vi "XYZ Ultrasonic Scanning Software v1.3 (Movement).vi"() -> ()   [LabVIEW 2020]
uses:
  <instrlib>/Arcus Ethernet Driver 1.0.0/ArcusEthernetComm/classes/Controller/_Controller.lvclass
panel:
  in  "Tab Control":T1(tab)
  in  "Check Rig Connection":bool
  out "Succesful Rig Connection":bool=TRUE
  in  "Error In":errorcluster
  in  "Move Y Distance":dbl
  in  "Set Starting Position":bool
  in  "Z Direction":bool=TRUE
  in  "Y Direction":bool=TRUE
  in  "Move X Distance":dbl
  in  "Move Z Distance":dbl
  in  "X Direction":bool=TRUE
  in  "Return To Home":bool
  in  "Move":bool
  in  "Start A-Scan":bool
  in  "Start B-Scan":bool
  in  "Initial X Direction":bool=TRUE
  in  "Initial Y Direction":bool=TRUE
  in  "Initial Z Direction":bool=TRUE
  in  "Confirm Scanning Parameters B-Scan":bool
  in  "Height (mm)":dbl
  in  "Width (mm)":dbl
  in  "Length (mm)":dbl
  in  "Select Axis To Scan":enum32{"No Selection", "X", "Y", "Z"}(radio)
  in  "Scan C-Scan":bool
  in  "Length (mm)":dbl
  in  "Width (mm)":dbl
  in  "Height (mm)":dbl
  in  "Confirm Dimensions":bool
  in  "Initial X Direction":bool=TRUE
  in  "Initial Y Direction":bool=TRUE
  in  "Initial Z Direction":bool=TRUE
  in  "Select Plane To Scan":enum32{"No Selection", "XY", "XZ", "YZ"}(radio)
  # "Moving To Starting Point (mm)"
  # "Scanning Parameters"
  # "Tank Dimensions"
  # "Y - Width"
  # "X - Length"
  # "Z - Height"
  # "Scanning Parameters"
  # "Tank Dimensions"
  # "Y - Width"
  # "X - Length"
  # "Z - Height"
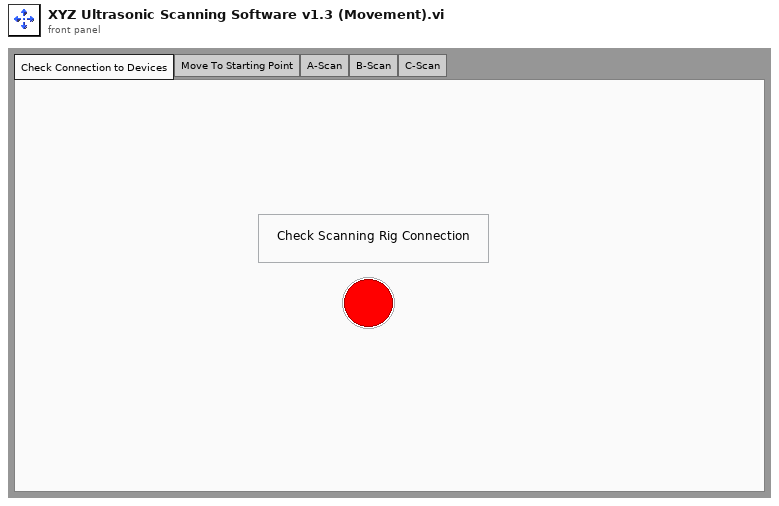
[diagram p1: front panel]
types:
  T1 = enum32{"Check Connection to Devices", "Move To Starting Point", "A-Scan", "B-Scan", "C-Scan"}
  T2 = enum8{"Enabled", "Disabled", "Disabled and Grayed Out"}
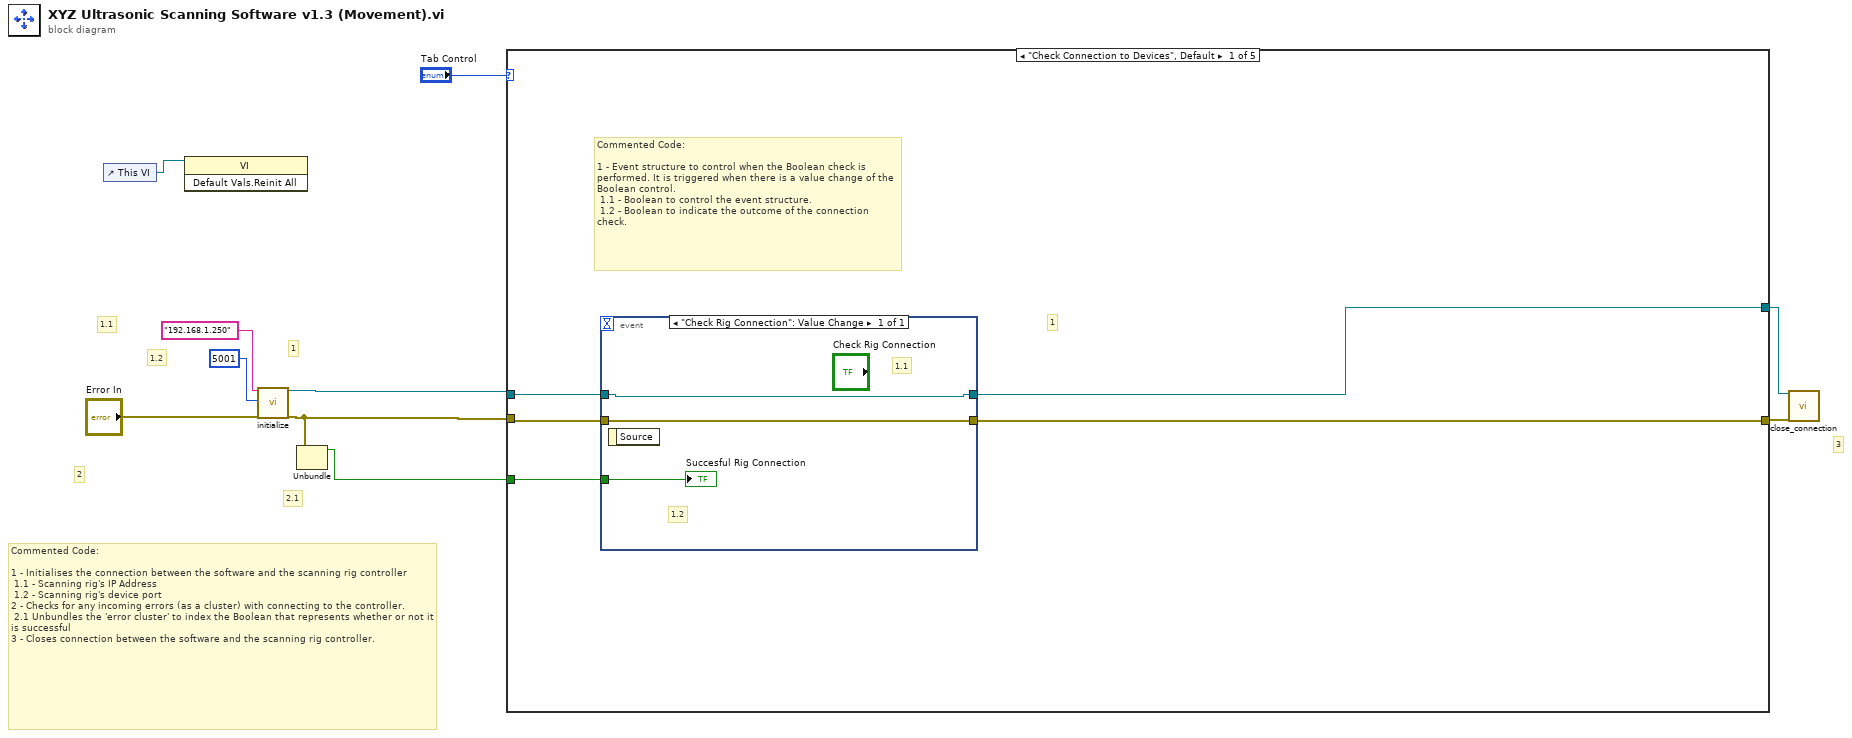
[diagram p0: block diagram]
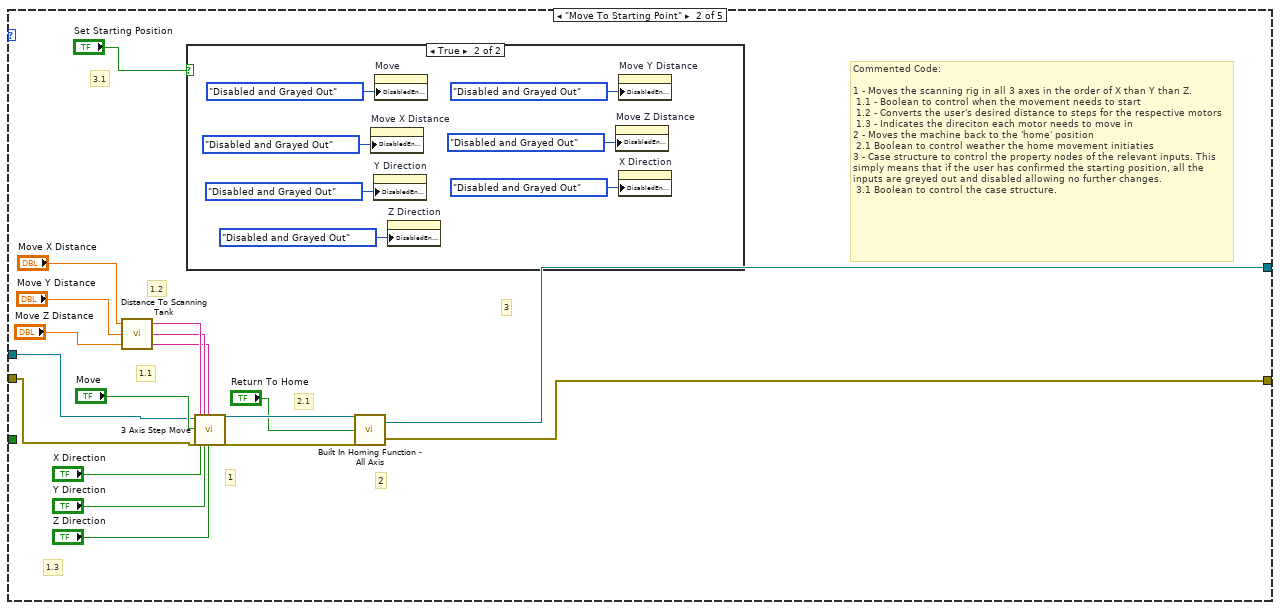
[diagram p2: hidden frame]
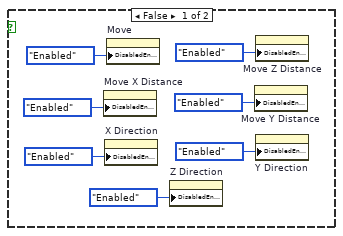
[diagram p3: hidden frame]
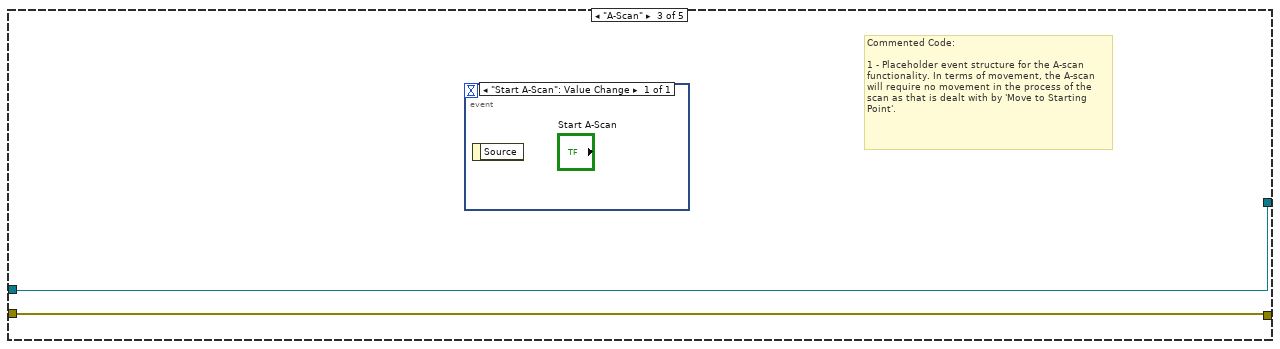
[diagram p4: hidden frame]
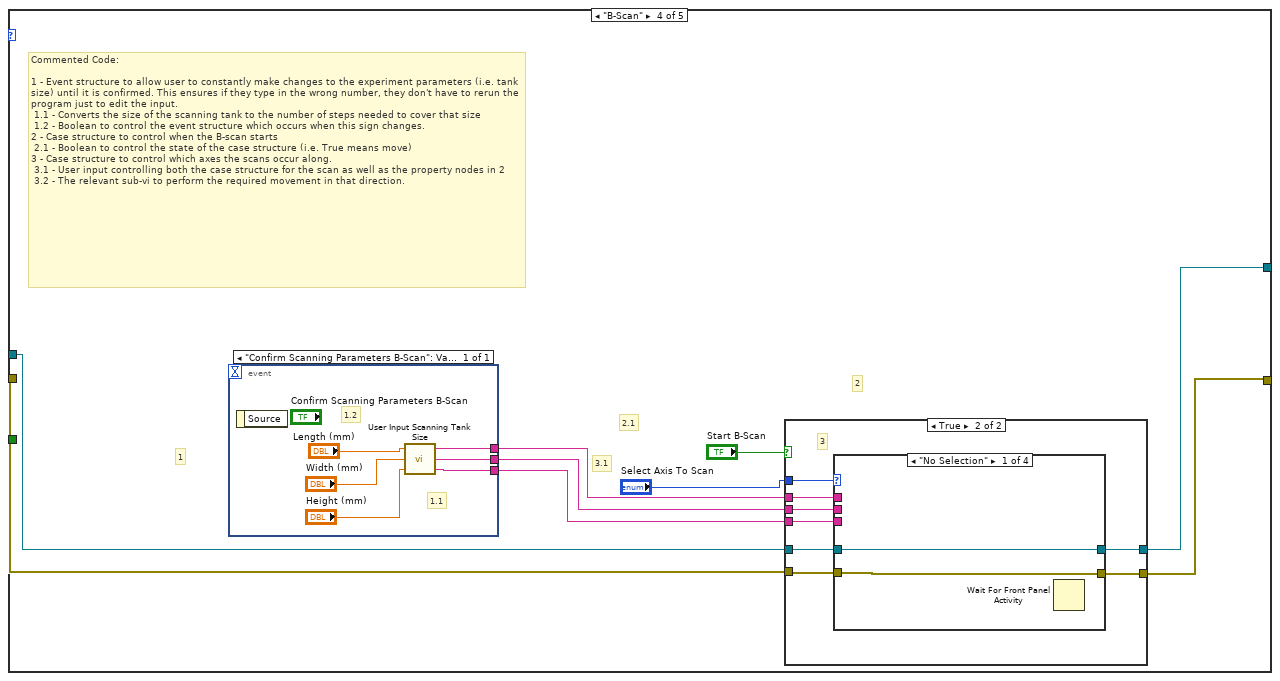
[diagram p5: hidden frame]
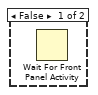
[diagram p6: hidden frame]
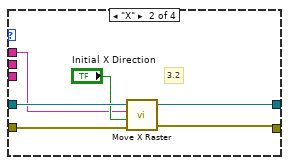
[diagram p7: hidden frame]
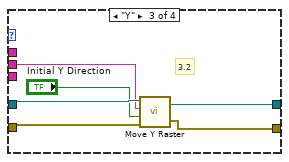
[diagram p8: hidden frame]
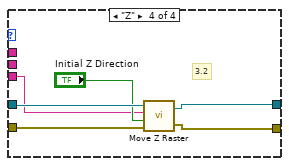
[diagram p9: hidden frame]
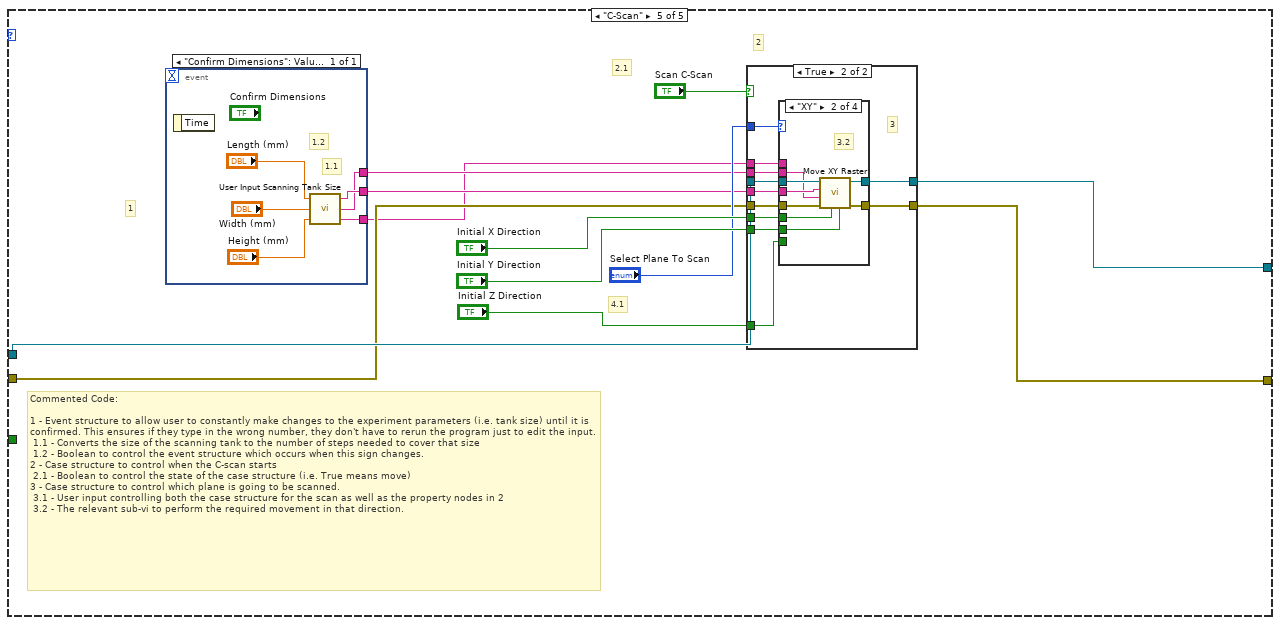
[diagram p10: hidden frame]
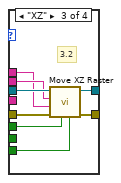
[diagram p13: hidden frame]
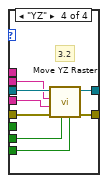
[diagram p14: hidden frame]
diagram:
  # "3"
  # "2"
  # "2.1"
  # "1.2"
  # "1.1"
  # "1"
  # "Commented Code:\n\n1 - Initialises the connection between the software and the scanning rig controller\n 1.1 - Scanning rig's IP Address\n 1.2 - Scanning rig's device port\n2 - Checks for any incoming errors (as a cluster) with connecting to the controller.  \n 2.1 Unbundles the 'error cluster' to index the Boolean that represents whether or not it is successful\n3 - Closes connection between the software and the scanning rig controller."
  n1 = control-ref of="This VI"() -> (w3:refnum<vi>)
  n2 = invoke class="VI" method="Default Vals.Reinit All"(reference=w3) -> ()  [unwired: 2 in, 3 out]
  n3 = call <instrlib>:"initialize.vi"("ip_address (in)"="192.168.1.250", "dev_port(def=5001)"=u16 5001, "error in (no error)"="Error In") -> ("reference (out)"=w9:refnum<class "_Controller.lvclass">, "error out"=w10:errorcluster)  [unwired: 15 in]
  n4 = Unbundle(w10) -> ("status"=w1:bool)  [unwired: 2 out]
  n5 = case shown="\"Check Connection to Devices\", Default" "Tab Control" {
    tunnel: w9 -> [w15 w26 w52 w60 w104]
    tunnel: [w13 w21 w52 w55 w103] -> w5
    tunnel: [w12 w22 w51 w53 w102] -> w4
    tunnel: w10 -> [w14 w25 w51 w59 w99]
    tunnel: w1 -> [w11 _ _ _ _]
    frame "Check Connection to Devices", Default {
      # "1"
      # "Commented Code:\n\n1 - Event structure to control when the Boolean check is performed. It is triggered when there is a value change of the Boolean control. \n 1.1 - Boolean to control the event structure. \n 1.2 - Boolean to indicate the outcome of the connection check."
      n6 = event shown="[0] \"Check Rig Connection\": Value Change" {
        selector: _ -> [_]
        dyn-events: _ -> [_]
        timeout: _ -> [_]
        tunnel: w15 -> [w18]
        tunnel: w14 -> [w17]
        tunnel: [w18] -> w13
        tunnel: [w17] -> w12
        tunnel: w11 -> [w16]
        event "Check Rig Connection": Value Change {
          # "1.1"
          # "1.2"
          n7 = event-data() -> ()  [unwired: 1 in, 1 out]
          "Succesful Rig Connection" <- w16
        }
      }
    }
    frame "Move To Starting Point" {
      # "3.1"
      # "3"
      # "2.1"
      # "2"
      # "1.3"
      # "1.1"
      # "1"
      # "1.2"
      # "Commented Code:\n\n1 - Moves the scanning rig in all 3 axes in the order of X than Y than Z.\n 1.1 - Boolean to control when the movement needs to start\n 1.2 - Converts the user's desired distance to steps for the respective motors\n 1.3 - Indicates the direciton each motor needs to move in\n2 - Moves the machine back to the 'home' position\n 2.1 Boolean to control weather the home movement initiaties \n3 - Case structure to control the property nodes of the relevant inputs. This simply means that if the user has confirmed the starting position, all the inputs are greyed out and disabled allowing no further changes.\n 3.1 Boolean to control the case structure."
      n8 = call "Distance To Scanning Tank.vi"("Move Z Distance (mm)"="Move Z Distance", "Move Y Distance (mm)"="Move Y Distance", "Move X Distance (mm)"="Move X Distance") -> ("Z Steps"=w34:string, "Y Steps"=w35:string, "X Steps"=w36:string)
      n9 = case shown="True" "Set Starting Position" {
        frame False {
          n10 = property on="Move X Distance" class="DigNum (strict)"("DisabledEnum"=T2."Enabled" ("Disabled")) -> ()  [unwired: 2 in, 2 out]
          n11 = property on="X Direction" class="Bool (strict)"("DisabledEnum"=T2."Enabled" ("Disabled")) -> ()  [unwired: 2 in, 2 out]
          n12 = property on="Move" class="Bool"("DisabledEnum"=T2."Enabled" ("Disabled")) -> ()  [unwired: 2 in, 2 out]
          n13 = property on="Z Direction" class="Bool (strict)"("DisabledEnum"=T2."Enabled" ("Disabled")) -> ()  [unwired: 2 in, 2 out]
          n14 = property on="Move Y Distance" class="DigNum (strict)"("DisabledEnum"=T2."Enabled" ("Disabled")) -> ()  [unwired: 2 in, 2 out]
          n15 = property on="Move Z Distance" class="DigNum (strict)"("DisabledEnum"=T2."Enabled" ("Disabled")) -> ()  [unwired: 2 in, 2 out]
          n16 = property on="Y Direction" class="Bool (strict)"("DisabledEnum"=T2."Enabled" ("Disabled")) -> ()  [unwired: 2 in, 2 out]
        }
        frame True {
          n17 = property on="Move X Distance" class="DigNum (strict)"("DisabledEnum"=T2."Disabled and Grayed Out" ("Disabled")) -> ()  [unwired: 2 in, 2 out]
          n18 = property on="Y Direction" class="Bool (strict)"("DisabledEnum"=T2."Disabled and Grayed Out" ("Disabled")) -> ()  [unwired: 2 in, 2 out]
          n19 = property on="Move" class="Bool"("DisabledEnum"=T2."Disabled and Grayed Out" ("Disabled")) -> ()  [unwired: 2 in, 2 out]
          n20 = property on="Z Direction" class="Bool (strict)"("DisabledEnum"=T2."Disabled and Grayed Out" ("Disabled")) -> ()  [unwired: 2 in, 2 out]
          n21 = property on="Move Z Distance" class="DigNum (strict)"("DisabledEnum"=T2."Disabled and Grayed Out" ("Disabled")) -> ()  [unwired: 2 in, 2 out]
          n22 = property on="Move Y Distance" class="DigNum (strict)"("DisabledEnum"=T2."Disabled and Grayed Out" ("Disabled")) -> ()  [unwired: 2 in, 2 out]
          n23 = property on="X Direction" class="Bool (strict)"("DisabledEnum"=T2."Disabled and Grayed Out" ("Disabled")) -> ()  [unwired: 2 in, 2 out]
        }
      }
      n24 = call "3 Axis Step Move.vi"("Reference In"=w26, "Move"="Move", "Error In"=w25, "X Steps"=w36, "Direction X"="X Direction", "Y Steps"=w35, "Direction Y"="Y Direction", "Z Steps"=w34, "Direcition Z"="Z Direction") -> ("Reference Out"=w24:refnum<class "_Controller.lvclass">, "Error Out"=w20:errorcluster)  [unwired: 17 in]
      n25 = call "Built In Homing Function - All Axis.vi"("Error In"=w20, "Home"="Return To Home", "Reference In"=w24) -> ("Error Out"=w22:errorcluster, "Reference Out"=w21:refnum<class "_Controller.lvclass">)
    }
    frame "A-Scan" {
      # "Commented Code:\n\n1 - Placeholder event structure for the A-scan functionality. In terms of movement, the A-scan will require no movement in the process of the scan as that is dealt with by 'Move to Starting Point'."
      n26 = event shown="[0] \"Start A-Scan\": Value Change" {
        selector: _ -> [_]
        dyn-events: _ -> [_]
        timeout: _ -> [_]
        event "Start A-Scan": Value Change {
          n27 = event-data() -> ()  [unwired: 1 in, 1 out]
        }
      }
    }
    frame "B-Scan" {
      # "3.1"
      # "2.1"
      # "2"
      # "1"
      # "Commented Code:\n\n1 - Event structure to allow user to constantly make changes to the experiment parameters (i.e. tank size) until it is confirmed. This ensures if they type in the wrong number, they don't have to rerun the program just to edit the input.\n 1.1 - Converts the size of the scanning tank to the number of steps needed to cover that size\n 1.2 - Boolean to control the event structure which occurs when this sign changes.\n2 - Case structure to control when the B-scan starts\n 2.1 - Boolean to control the state of the case structure (i.e. True means move) \n3 - Case structure to control which axes the scans occur along. \n 3.1 - User input controlling both the case structure for the scan as well as the property nodes in 2\n 3.2 - The relevant sub-vi to perform the required movement in that direction."
      n28 = event shown="[0] \"Confirm Scanning Parameters B-Scan\": Value Change" {
        selector: _ -> [_]
        dyn-events: _ -> [_]
        timeout: _ -> [_]
        tunnel: [w92] -> w56
        tunnel: [w91] -> w57
        tunnel: [w90] -> w58
        event "Confirm Scanning Parameters B-Scan": Value Change {
          # "1.2"
          # "1.1"
          n29 = event-data() -> ()  [unwired: 1 in, 1 out]
          n30 = call "User Input Scanning Tank Size.vi"("Height (mm)"="Height (mm)", "Width (mm)"="Width (mm)", "Length (mm)"="Length (mm)") -> ("Z Steps"=w92:string, "Y Steps"=w91:string, "X Steps"=w90:string)
        }
      }
      n31 = case shown="True" "Start B-Scan" {
        tunnel: "Select Axis To Scan" -> [_ w69]
        tunnel: w60 -> [_ w68]
        tunnel: w59 -> [_ w62]
        tunnel: w58 -> [_ w67]
        tunnel: w57 -> [_ w66]
        tunnel: w56 -> [_ w65]
        tunnel: [_ w64] -> w53
        tunnel: [_ w63] -> w55
        frame False {
          n32 = Wait For Front Panel Activity() -> ()  [unwired: 3 in, 1 out]
        }
        frame True {
          # "3"
          n33 = case shown="\"No Selection\"" w69 {
            tunnel: w68 -> [w71 w77 w83 w89]
            tunnel: w62 -> [w70 w74 w82 w88]
            tunnel: [w70 w72 w78 w84] -> w64
            tunnel: w67 -> [_ w75 _ _]
            tunnel: w66 -> [_ _ w80 _]
            tunnel: w65 -> [_ _ _ w86]
            tunnel: [w71 w73 w79 w85] -> w63
            frame "No Selection" {
              n34 = Wait For Front Panel Activity() -> ()  [unwired: 3 in, 1 out]
            }
            frame "X" {
              # "3.2"
              n35 = call "Move X Raster.vi"("Error In"=w74, "Initial Direction"="Initial X Direction", "X Number of Steps"=w75, "Reference In"=w77) -> ("Error Out"=w72:errorcluster, "Reference Out"=w73:refnum<class "_Controller.lvclass">)  [unwired: 1 in]
            }
            frame "Y" {
              # "3.2"
              n36 = call "Move Y Raster.vi"("Error In"=w82, "Initial Direction"="Initial Y Direction", "Y Number of Steps"=w80, "Refernce In"=w83) -> ("Error Out"=w78:errorcluster, "Reference Out"=w79:refnum<class "_Controller.lvclass">)
            }
            frame "Z" {
              # "3.2"
              n37 = call "Move Z Raster.vi"("Error In"=w88, "Initial Direction"="Initial Z Direction", "Z Number of Steps"=w86, "Reference In"=w89) -> ("Error Out"=w84:errorcluster, "Reference Out"=w85:refnum<class "_Controller.lvclass">)
            }
          }
        }
      }
    }
    frame "C-Scan" {
      # "4.1"
      # "2.1"
      # "2"
      # "1"
      # "Commented Code:\n\n1 - Event structure to allow user to constantly make changes to the experiment parameters (i.e. tank size) until it is confirmed. This ensures if they type in the wrong number, they don't have to rerun the program just to edit the input.\n 1.1 - Converts the size of the scanning tank to the number of steps needed to cover that size\n 1.2 - Boolean to control the event structure which occurs when this sign changes. \n2 - Case structure to control when the C-scan starts\n 2.1 - Boolean to control the state of the case structure (i.e. True means move) \n3 - Case structure to control which plane is going to be scanned. \n 3.1 - User input controlling both the case structure for the scan as well as the property nodes in 2\n 3.2 - The relevant sub-vi to perform the required movement in that direction."
      n38 = event shown="[0] \"Confirm Dimensions\": Value Change" {
        selector: _ -> [_]
        dyn-events: _ -> [_]
        timeout: _ -> [_]
        tunnel: [w145] -> w98
        tunnel: [w144] -> w97
        tunnel: [w143] -> w96
        event "Confirm Dimensions": Value Change {
          # "1.1"
          # "1.2"
          n39 = event-data() -> ()  [unwired: 1 in, 1 out]
          n40 = call "User Input Scanning Tank Size.vi"("Height (mm)"="Height (mm)", "Width (mm)"="Width (mm)", "Length (mm)"="Length (mm)") -> ("Z Steps"=w143:string, "Y Steps"=w144:string, "X Steps"=w145:string)
        }
      }
      n41 = case shown="True" "Scan C-Scan" {
        tunnel: "Select Plane To Scan" -> [_ w118]
        tunnel: "Initial X Direction" -> [_ w117]
        tunnel: "Initial Y Direction" -> [_ w116]
        tunnel: "Initial Z Direction" -> [_ w115]
        tunnel: w104 -> [_ w114]
        tunnel: w99 -> [_ w113]
        tunnel: [_ w112] -> w103
        tunnel: [_ w111] -> w102
        tunnel: w98 -> [_ w110]
        tunnel: w97 -> [_ w109]
        tunnel: w96 -> [_ w108]
        frame False {
        }
        frame True {
          # "3"
          n42 = case shown="\"XY\"" w118 {
            tunnel: w117 -> [_ w122 w130 _]
            tunnel: w116 -> [_ w121 _ w138]
            tunnel: w115 -> [_ _ w129 w137]
            tunnel: w114 -> [_ w126 w131 w142]
            tunnel: w113 -> [_ w125 w132 w141]
            tunnel: [_ w124 w134 w140] -> w112
            tunnel: [_ w123 w133 w139] -> w111
            tunnel: w110 -> [_ w120 _ w135]
            tunnel: w109 -> [_ w119 w128 w136]
            tunnel: w108 -> [_ _ w127 _]
            frame "No Selection", Default {
            }
            frame "XY" {
              # "3.2"
              n43 = call "Move XY Raster.vi"("Initial Y Direction"=w121, "Initial X Direction"=w122, "Error In"=w125, "Y Number of Steps"=w119, "X Number of Steps"=w120, "Reference In"=w126) -> ("Error Out"=w123:errorcluster, "Reference Out"=w124:refnum<class "_Controller.lvclass">)  [unwired: 4 in]
            }
            frame "XZ" {
              # "3.2"
              n44 = call "Move XZ Raster.vi"("Initial Z Direction"=w129, "Initial X Direction"=w130, "Error In"=w132, "Z Number of Steps"=w127, "X Number of Steps"=w128, "Reference In"=w131) -> ("Error Out"=w133:errorcluster, "Reference Out"=w134:refnum<class "_Controller.lvclass">)  [unwired: 4 in]
            }
            frame "YZ" {
              # "3.2"
              n45 = call "Move YZ Raster.vi"("Initial Z Direction"=w137, "Initial Y Direction"=w138, "Error In"=w141, "Z Number of Steps"=w135, "Y Number of Steps"=w136, "Reference In"=w142) -> ("Error Out"=w139:errorcluster, "Reference Out"=w140:refnum<class "_Controller.lvclass">)  [unwired: 4 in]
            }
          }
        }
      }
    }
  }
  n46 = call <instrlib>:"close_connection.vi"("reference (in)"=w5, "error in (no error)"=w4) -> ()  [unwired: 16 in, 2 out]
